vi "MAIN_auto_2chan.vi"() -> ()   [LabVIEW 2017]
uses:
  <vilib>/Utility/file.llb/Write Delimited Spreadsheet (string).vi
panel:
  in  "Tab Control":enum32{"Controles", "Canales", "juntos"}(tab)
  in  "Archivos de\nreferencias (.csv)":path=path "D:/Registros_de_rodadura/ENE_2020/Ene_2020_out/02_total_reff"
  out "filenames":string[](array[string])
  out "csvs de referencia)":i32
  out "last\nconcatenated string":string
  in  "Archivos de \nfeatures (.csv)":path=path "D:/Registros_de_rodadura/ENE_2020/Ene_2020_out/04_FEATS_tercio_2chan"
  in  "Referencias de TDMSs":path=path "D:/Registros_de_rodadura/ENE_2020/Ene_2020_in/TDMS&GPX"
  out "All Files in Dir":path[](array[path])
  out "tdms":i32
  in  "Largo de ventada \ntemporal en N samples":dbl=44100.0
  in  "Canal 1":string[](array[string])=["cDAQ1Mod1_ai0"]
  in  "frequency range":T1={"low band"=enum."20 Hz", "high band"=enum."20000 Hz"}
  out "Numeric":i32
  in  "Canal 2":string[](array[string])=["cDAQ1Mod1_ai0"]
  out "chan1":string[][](array[string]) caption="TO CSV chan 1."
  out "chan2":string[][](array[string]) caption="TO CSV chan 2."
  out "output array":string[][](array[string])
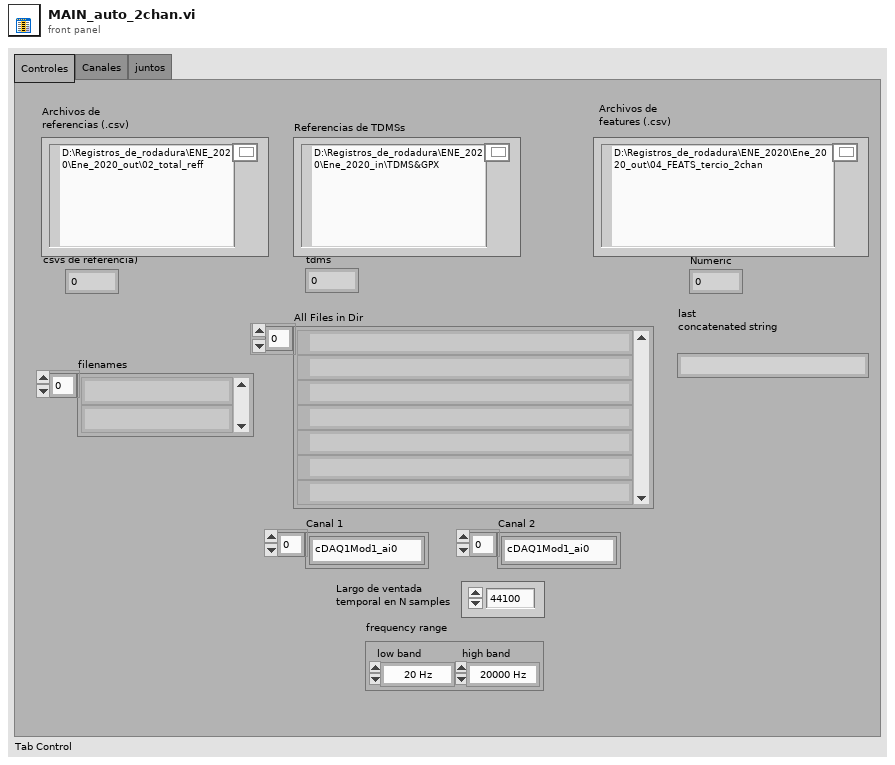
[diagram p1: front panel]
types:
  T1 = cluster{"low band":enum16{"20 Hz", "25 Hz", "31.5 Hz", "40 Hz", "50 Hz", "63 Hz", "80 Hz", "100 Hz", "125 Hz", "160 Hz", "200 Hz", "250 Hz", "315 Hz", "400 Hz", "500 Hz", "630 Hz", "800 Hz", "1000 Hz", "1250 Hz", "1600 Hz", "2000 Hz", "2500 Hz", "3150 Hz", "4000 Hz", "5000 Hz", "6300 Hz", "8000 Hz", "10000 Hz", "12500 Hz", "16000 Hz", "20000 Hz"}, "high band":enum16{"20 Hz", "25 Hz", "31.5 Hz", "40 Hz", "50 Hz", "63 Hz", "80 Hz", "100 Hz", "125 Hz", "160 Hz", "200 Hz", "250 Hz", "315 Hz", "400 Hz", "500 Hz", "630 Hz", "800 Hz", "1000 Hz", "1250 Hz", "1600 Hz", "2000 Hz", "2500 Hz", "3150 Hz", "4000 Hz", "5000 Hz", "6300 Hz", "8000 Hz", "10000 Hz", "12500 Hz", "16000 Hz", "20000 Hz"}}
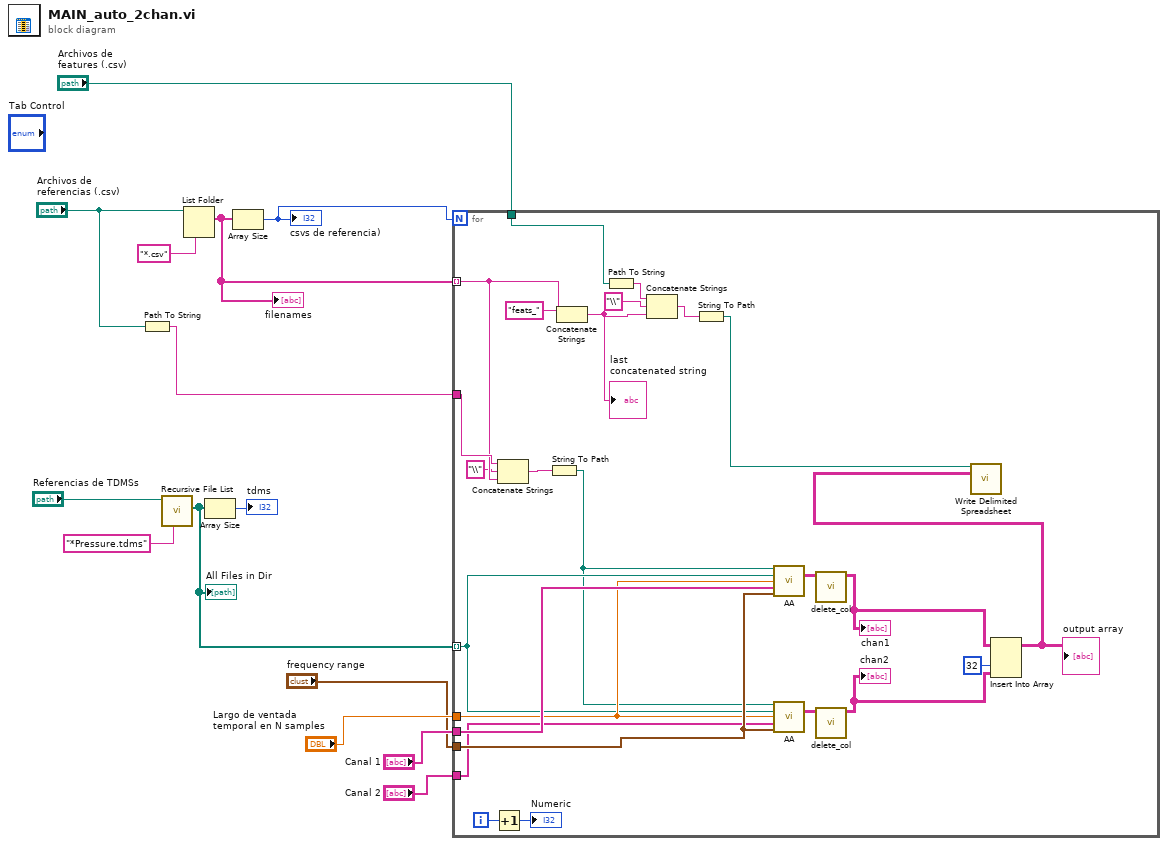
[diagram p0: block diagram]
diagram:
  n1 = Path To String(path="Archivos de\nreferencias (.csv)") -> (string=w6:string)
  n2 = call <vilib>:"Recursive File List.vi"("pattern"="*Pressure.tdms", "Folder Path"="Referencias de TDMSs") -> ("All Files in Dir"=w9:path[])  [unwired: 5 in, 4 out]
  "All Files in Dir" <- w9
  n3 = List Folder(path="Archivos de\nreferencias (.csv)", pattern="*.csv") -> (filenames=w8:string[])  [unwired: 2 in, 3 out]
  "filenames" <- w8
  n4 = Array Size(array=w9) -> (size(s)=→"tdms":i32)
  n5 = Array Size(array=w8) -> (size(s)=w2:i32)
  "csvs de referencia)" <- w2
  n6 = for {
    N: w2 -> [_]
    tunnel: w8 -> [w32] mode=indexing
    tunnel: "Archivos de \nfeatures (.csv)" -> [w30]
    tunnel: w9 -> [w23] mode=indexing
    tunnel: w6 -> [w34]
    tunnel: "Largo de ventada \ntemporal en N samples" -> [w24]
    tunnel: "Canal 1" -> [w29]
    tunnel: "frequency range" -> [w26]
    tunnel: "Canal 2" -> [w25]
    i -> [w28]
    n7 = Increment(x=w28) -> (x+1=→"Numeric":i32)
    n8 = Concatenate Strings(w34, "\\" ("string"), w32) -> (w33:string)
    n9 = String To Path(string=w33) -> (path=w22:path)
    n10 = Concatenate Strings("feats_", w32) -> (w37:string)
    "last\nconcatenated string" <- w37
    n11 = Path To String(path=w30) -> (string=w38:string)
    n12 = Concatenate Strings(w38, "\\" ("string"), w37) -> (w35:string)
    n13 = String To Path(string=w35) -> (path=w15:path)
    n14 = call "AA.vi"("Archivo de\nreferencias (.csv)"=w22, "ARCHIVO\nTDMS"=w23, "Largo de ventada temporal en N samples"=w24, "Canal"=w29, "frequency range"=w26) -> ("TO CSV."=w21:string[][])  [unwired: 10 in]
    n15 = call "AA.vi"("Archivo de\nreferencias (.csv)"=w22, "ARCHIVO\nTDMS"=w23, "Largo de ventada temporal en N samples"=w24, "Canal"=w25, "frequency range"=w26) -> ("TO CSV."=w20:string[][])  [unwired: 10 in]
    n16 = call "delete_col.vi"("TO CSV. in"=w21) -> ("TO CSV. out"=w18:string[][])  [unwired: 9 in, 1 out]
    "chan1" <- w18
    n17 = call "delete_col.vi"("TO CSV. in"=w20) -> ("TO CSV. out"=w17:string[][])  [unwired: 9 in, 1 out]
    "chan2" <- w17
    n18 = Insert Into Array(array=w18, index (col)=32 ("disabled index (col)"), new element=w17) -> (w16:string[][])  [unwired: 1 in]
    "output array" <- w16
    n19 = call-poly <vilib>:"Write Delimited Spreadsheet.vi"("file path (dialog if empty)"=w15, "2D data"=w16) -> ()  [unwired: 12 in, 2 out]
  }
